vi "Save File Create Station Specific File Name.vi"(8 "Error In":errorcluster, 10 "Station ID":string, 11 "Tool Base Path":path) -> (0 "Error Out":errorcluster, 2 "RLT Backup Data Path":path, 3 "Station Specific Configuration File":path)   [LabVIEW 2019]
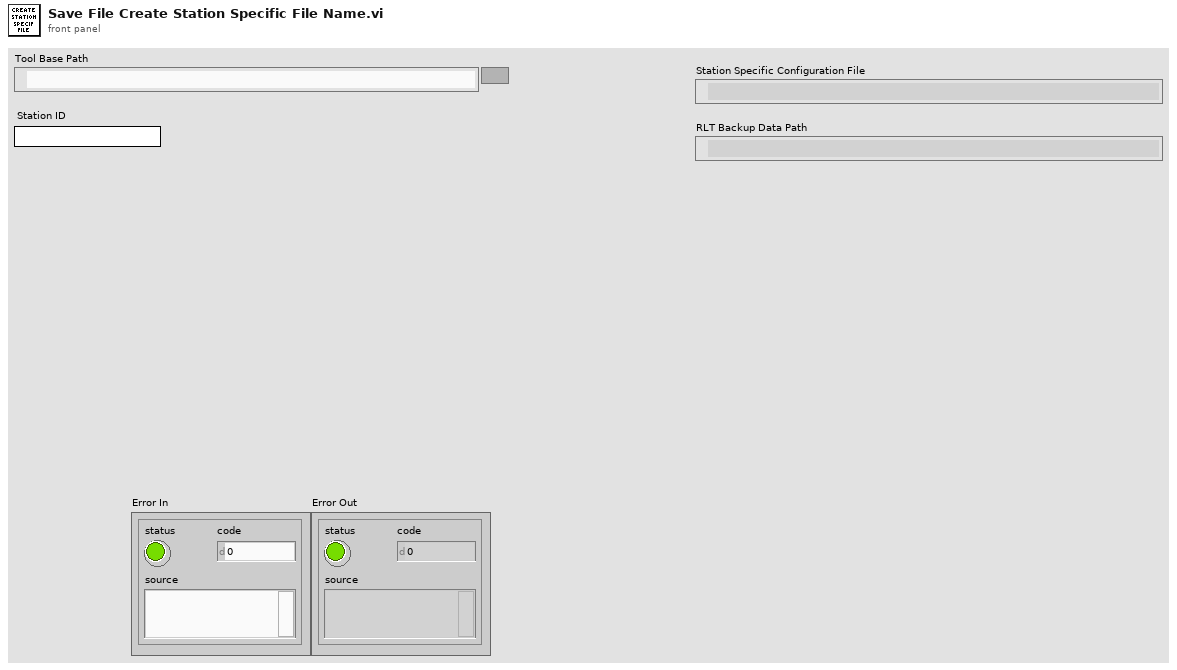
[diagram p1: front panel]
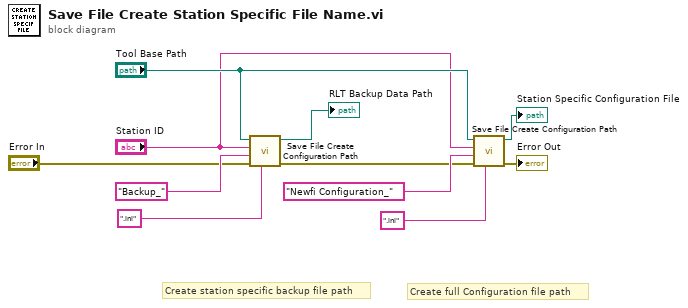
[diagram p0: block diagram]
diagram:
  # "Create full Configuration file path"
  # "Create station specific backup file path"
  n1 = call "Save File Create Configuration Path.vi"("File Type (.ini)"=".ini", "Error In"="Error In", "Configuration Name"="Backup_" ("name or relative path"), "Station ID"="Station ID", "Tool Base Path"="Tool Base Path") -> ("Error Out"=w4:errorcluster, "New Configuration File Path"=→"RLT Backup Data Path":path)  [unwired: 5 in]
  n2 = call "Save File Create Configuration Path.vi"("File Type (.ini)"=".ini", "Error In"=w4, "Configuration Name"="Newfi Configuration_", "Station ID"="Station ID", "Tool Base Path"="Tool Base Path") -> ("Error Out"=→"Error Out":errorcluster, "New Configuration File Path"=→"Station Specific Configuration File":path)  [unwired: 5 in]
